vi "FTW-Container-Destroy.vi"(0 "Container":refnum<class "FTW-Container.lvclass">, 11 "error in":errorcluster) -> (15 "error out":errorcluster)   [LabVIEW 2014, in "FTW-Container.lvclass"]
uses:
  FTW-Container.lvclass
panel:
  # "Inputs"
  # "Outputs"
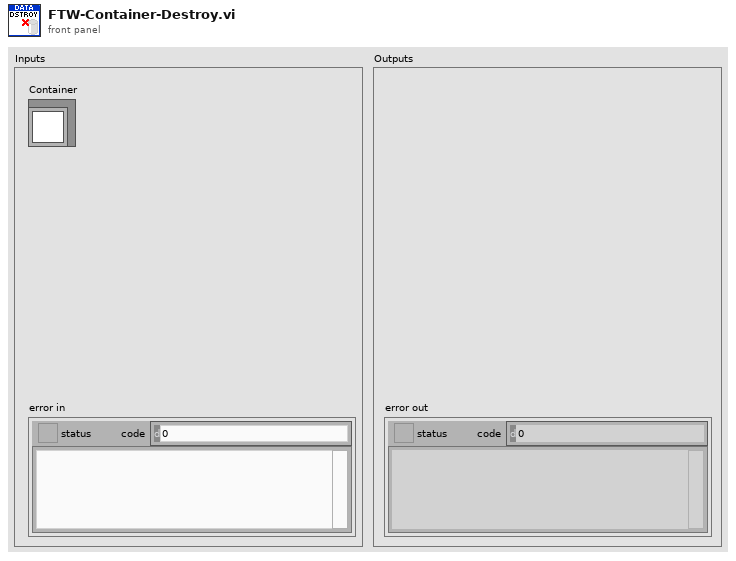
[diagram p1: front panel]
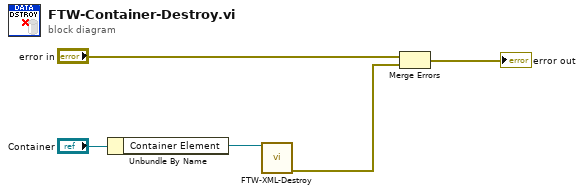
[diagram p0: block diagram]
diagram:
  n1 = Unbundle By Name("Container") -> ("Container Element"=w2:refnum<k20>)
  n2 = call "FTW-XML-Destroy.vi"("XML Node"=w2) -> ("error out"=w1:errorcluster)  [unwired: 14 in]
  n3 = Merge Errors("error in", w1) -> (→"error out":errorcluster)
